vi "火灾报警系统设计.vi"() -> ()   [LabVIEW 2018]
panel:
  in  "结束":bool
  out "报警灯":bool
  in  "紫外输入":bool
  in  "温感输入":bool
  in  "烟感输入":bool
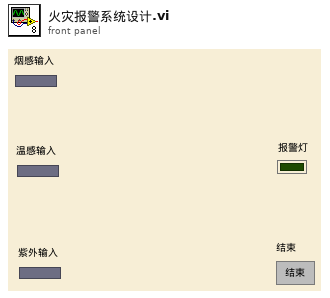
[diagram p1: front panel]
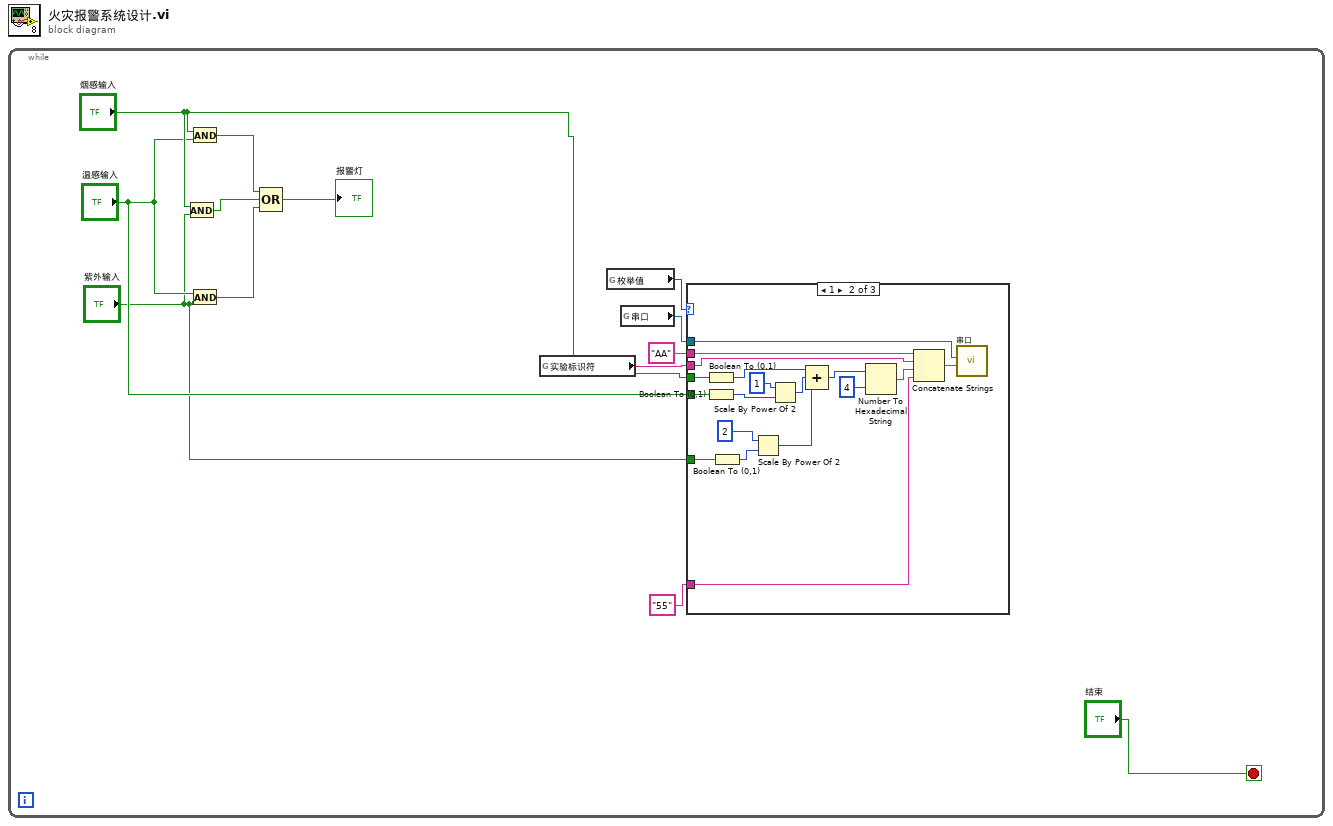
[diagram p0: block diagram]
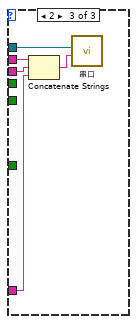
[diagram p3: hidden frame]
diagram:
  n1 = while {
    stop <- "结束" stop-if-true
    n2 = And(x="烟感输入", y="紫外输入") -> (x .and. y?=w12:bool)
    n3 = And(x="烟感输入", y="温感输入") -> (x .and. y?=w13:bool)
    n4 = And(x="温感输入", y="紫外输入") -> (x .and. y?=w11:bool)
    n5 = Compound Arithmetic op=OR ("复合运算")(w13, w12, w11) -> (→"报警灯":bool)
    n6 = global read "全局变量.vi" "实验标识符"() -> (w6:string)
    n7 = global read "全局变量.vi" "枚举值"() -> (w8:i8)
    n8 = global read "全局变量.vi" "串口"() -> (w7:refnum<visa-resource-name>)
    n9 = case shown="1" w8 {
      tunnel: "温感输入" -> [_ w26 _]
      tunnel: "烟感输入" -> [_ w25 _]
      tunnel: w7 -> [_ w24 w34]
      tunnel: w6 -> [_ w23 w35]
      tunnel: "55" -> [_ w22 w32]
      tunnel: "AA" -> [_ w21 w33]
      tunnel: "紫外输入" -> [_ w15 _]
      frame 0, Default {
      }
      frame 1 {
        n10 = Boolean To (0,1)(Boolean=w25) -> (0, 1=w30:i16)
        n11 = Boolean To (0,1)(Boolean=w26) -> (0, 1=w28:i16)
        n12 = Boolean To (0,1)(Boolean=w15) -> (0, 1=w16:i16)
        n13 = Scale By Power Of 2(n=2, x=w16) -> (x*2^n=w17:i16)
        n14 = Scale By Power Of 2(n=1, x=w28) -> (x*2^n=w29:i16)
        n15 = Compound Arithmetic op=ADD ("复合运算")(w30, w29, w17) -> (w20:i16)
        n16 = Number To Hexadecimal String(1:4, 2:w20) -> (0:w18:string)
        n17 = Concatenate Strings(w21, w23, w18, w22) -> (w31:string)
        n18 = call "串口.vi"("字符串"=w31, "VISA resource name"=w24) -> ()  [unwired: 10 in]
      }
      frame 2 {
        n19 = Concatenate Strings(w33, w35, w32) -> (w36:string)
        n20 = call "串口.vi"("字符串"=w36, "VISA resource name"=w34) -> ()  [unwired: 10 in]
      }
    }
  }
